vi "Timeout.vi"(8 "error in (no error)":errorcluster, 10 "allow send timeout":bool=TRUE, 11 "PolledDriver in":refnum<class "PolledDriver.lvclass">) -> (0 "error out":errorcluster, 2 "timed out?":bool, 3 "PolledDriver out":refnum<class "PolledDriver.lvclass">)   [LabVIEW 2013, in "PolledDriver.lvclass"]
doc: "Handles a timeout that occurs when an expected response to a message doesn't arrive on time. Tries to resend the message a fixed number of times"
uses:
  PolledDriver.lvclass
  BaseDriver/BaseDriver.lvclass
  PolledDriver.lvclass/PolledDriver.ctl
  response.ctl
  driver_status.ctl
  Responder/BaseResponder/BaseResponder.lvclass
  BaseDriver/Read Responder.vi
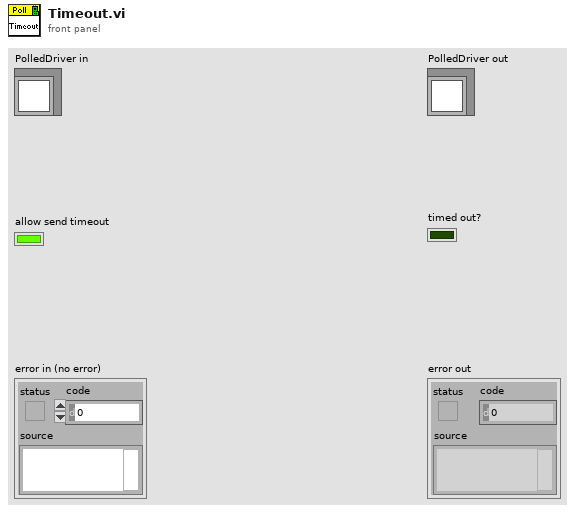
[diagram p1: front panel]
types:
  T1 = typedef "driver_status.ctl" = enum16{"Normal", "Startup", "Connection lost", "Reconnected", "Timeout", "Idle", "Busy"}
  T2 = typedef "response.ctl" = cluster{"driver status":T1, "Sender":string, "Type":i32, "Variant":variant}
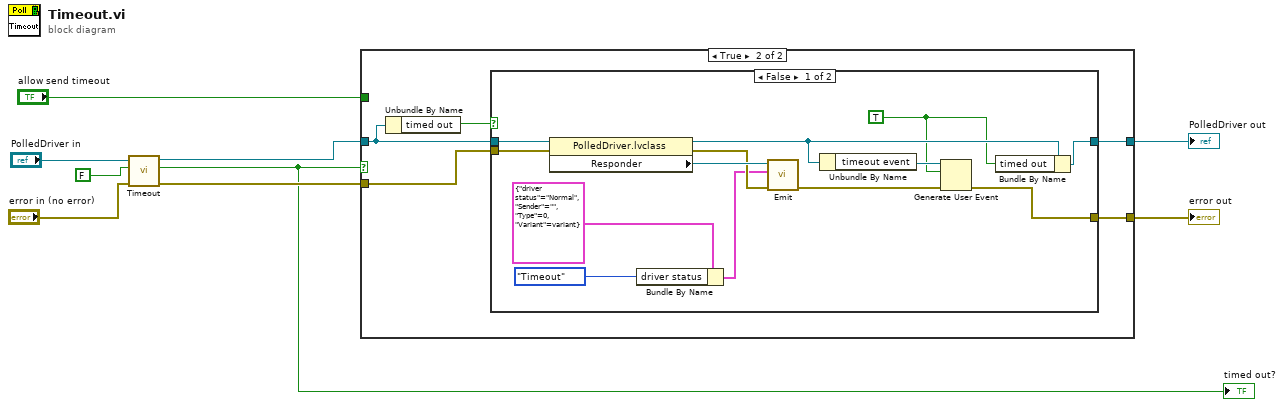
[diagram p0: block diagram]
diagram:
  n1 = call-parent "Timeout.vi"("error in (no error)"="error in (no error)", "allow send timeout"=FALSE, "BaseDriver in"="PolledDriver in") -> ("error out"=w4:errorcluster, "timed out?"=w3:bool, "BaseDriver out"=w5:refnum<class "PolledDriver.lvclass">)  [unwired: 6 in]
  "timed out?" <- w3
  n2 = case shown="True" w3 {
    tunnel: w5 -> [w11 w14]
    tunnel: [w11 w16] -> w9
    tunnel: [w10 w15] -> w8
    tunnel: w4 -> [w10 w12]
    tunnel: "allow send timeout" -> [_ _]
    frame False {
    }
    frame True {
      n3 = Unbundle By Name(w14) -> ("timed out"=w13:bool)
      n4 = case shown="False" w13 {
        tunnel: w12 -> [w28 w31]
        tunnel: [w26 w30] -> w16
        tunnel: [w17 w31] -> w15
        tunnel: w14 -> [w21 w30]
        frame False {
          w22 = TRUE ("timed out")
          n5 = property on="Property Node" class="PolledDriver.lvclass"(reference=w21, error in=w28) -> (reference out=w25:refnum<class "PolledDriver.lvclass">, error out=w27:errorcluster, "Responder"=w29:refnum<class "BaseResponder.lvclass">)
          n6 = Bundle By Name(cluster=T2 {"driver status"=enum."Normal", "Sender"="", "Type"=0, "Variant"=variant} ("response"), "driver status"=driver_status."Timeout") -> (w18:T2)
          n7 = call-dynamic "Emit.vi"("error in (no error)"=w27, "response"=w18, "BaseResponder in"=w29) -> ("error out"=w23:errorcluster)  [unwired: 7 in, 1 out]
          n8 = Unbundle By Name(w25) -> ("timeout event"=w24:refnum<user-event>)
          n9 = Generate User Event(user event=w24, event data cluster=w22, error in=w23) -> (error out=w17:errorcluster)  [unwired: 1 in, 1 out]
          n10 = Bundle By Name(cluster=w25, "timed out"=w22) -> (w26:refnum<class "PolledDriver.lvclass">)
        }
        frame True {
        }
      }
    }
  }
  "error out" <- w8
  "PolledDriver out" <- w9
